vi "SpeedAccelM1M2_2.vi"(4 "Accel2":u32 max=127 step=1, 5 "Speed2":i32 max=127 step=1, 6 "Accel1":u32 max=127 step=1, 7 "error in (no error)":errorcluster, 8 "Address":u8, 9 "Speed1":i32 max=127 step=1, 10 "VISA Refnum in":refnum<visa-resource-name>) -> (0 "error out":errorcluster, 2 "Valid":bool, 3 "VISA Refnum out":refnum<visa-resource-name>)   [LabVIEW 2015, in "Ion Motion Roboclaw.lvlib"]
uses:
  <instrlib>/Ion Motion Roboclaw/Ion Motion Roboclaw.lvlib
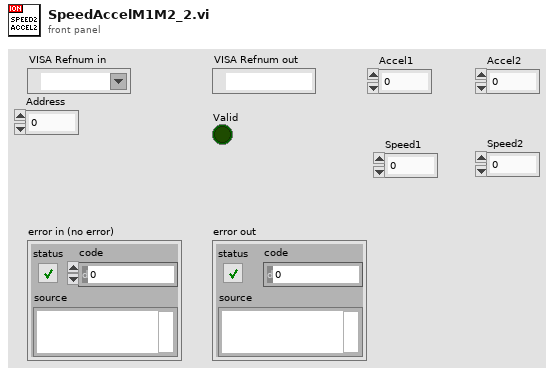
[diagram p1: front panel]
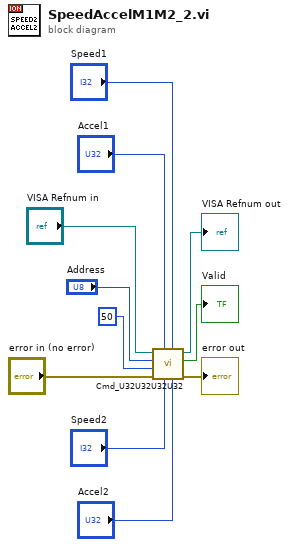
[diagram p0: block diagram]
diagram:
  n1 = call <instrlib>:"Cmd_U32U32U32U32.vi"("Arg3"="Accel2", "Arg2"="Speed1", "Arg4"="Speed2", "Arg1"="Accel1", "error in (no error)"="error in (no error)", "Cmd"=u8 50, "Address"="Address", "VISA Refnum in"="VISA Refnum in") -> ("error out"=→"error out":errorcluster, "Valid"=→"Valid":bool, "VISA Refnum out"=→"VISA Refnum out":refnum<visa-resource-name>)  [unwired: 1 in]
